vi "엔코드 속도(RPS) 측정.vi"() -> ()   [LabVIEW 2014]
uses:
  <vilib>/DAQmx/create/channels.llb/DAQmx Create Channel (CI-Position-Angular Encoder).vi
  <vilib>/DAQmx/read.llb/DAQmx Read (Counter DBL 1Chan 1Samp).vi
panel:
  out "RPS":dbl
  out "data":dbl caption="데이터" format="%0.2f"
  in  "정지":bool
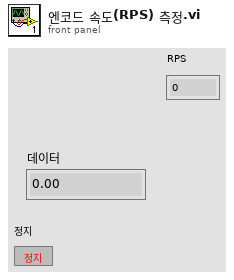
[diagram p1: front panel]
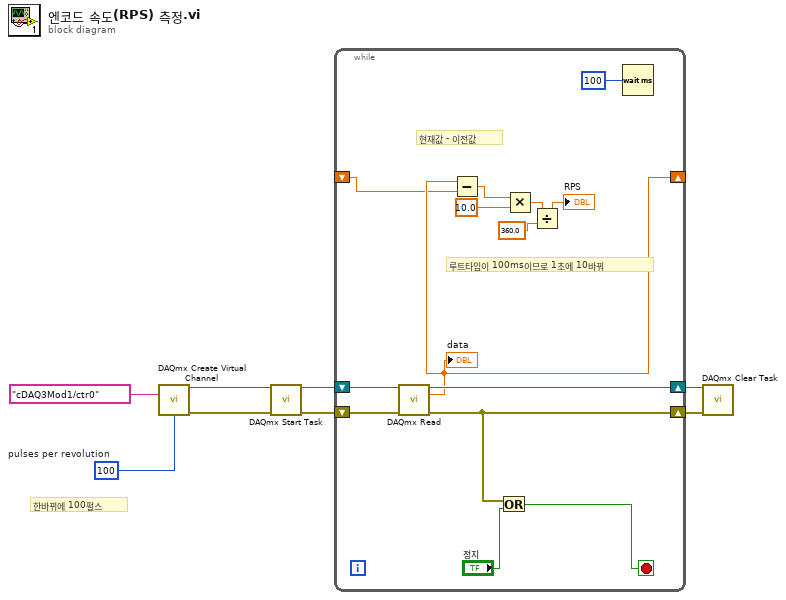
[diagram p0: block diagram]
diagram:
  w7 = u32 100  # pulses per revolution
  # "한바뀌에 100펄스"
  n1 = call-poly <vilib>:"DAQmx Create Virtual Channel.vi"("counter"=tag "cDAQ3Mod1/ctr0", "pulses per revolution"=w7) -> ("task out"=w6:refnum<k21>, "error out"=w5:errorcluster)  [unwired: 12 in]
  n2 = call <vilib>:"DAQmx Start Task.vi"("task/channels in"=w6, "error in"=w5) -> ("task out"=w4:refnum<k21>, "error out"=w3:errorcluster)  [unwired: 12 in]
  n3 = while {
    shift-right: [w20] -> w2
    shift-left: w4 -> [w22]
    shift-right: [w18] -> w1
    shift-left: w3 -> [w21]
    shift-right: [w15] -> _
    shift-left: _ -> [w14]
    stop <- w16 stop-if-true
    # "루트타임이 100ms이므로 1초에 10바꿔"
    # "현재값 - 이전값"
    n4 = call-poly <vilib>:"DAQmx Read.vi"("task/channels in"=w22, "error in"=w21) -> ("task out"=w20:refnum<k21>, "data"=w15:dbl, "error out"=w18:errorcluster)  [unwired: 11 in]
    "data" <- w15
    n5 = Subtract(x=w15, y=w14) -> (x-y=w13:dbl)
    n6 = Or(x=w18, y="정지") -> (x .or. y?=w16:bool)
    n7 = Multiply(x=w13, y=10.0) -> (x*y=w11:dbl)
    n8 = Divide(x=w11, y=360.0) -> (x/y=→"RPS":dbl)
    n9 = Wait (ms)(milliseconds to wait=u32 100 ("ms 배수")) -> ()  [unwired: 1 out]
  }
  n10 = call <vilib>:"DAQmx Clear Task.vi"("task in"=w2, "error in"=w1) -> ()  [unwired: 13 in, 1 out]
